vi "Save Recall Sweep List.vi"(8 "error in (no error)":errorcluster, 9 "File Name (\"\")":string, 10 "Sweep List Operation (0: Save)":u16(ring) items=["Save", "Recall"], 11 "VISA resource name":refnum<visa-resource-name>) -> (0 "error out":errorcluster, 3 "VISA resource name out":refnum<visa-resource-name>)   [LabVIEW 2009, in "Agilent PSG MXG Series.lvlib"]
doc: "Saves or recalls a sweep list to or from the file you specify."
uses:
  Agilent PSG MXG Series.lvlib
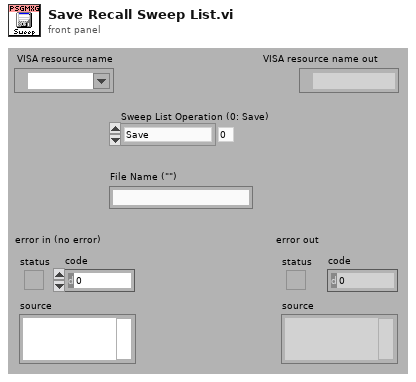
[diagram p1: front panel]
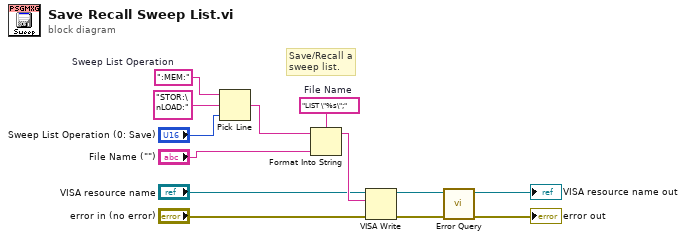
[diagram p0: block diagram]
diagram:
  w9 = "LIST \"%s\";"  # File Name
  w13 = ":MEM:"  # Sweep List Operation
  # "Save/Recall a\nsweep list."
  n1 = Pick Line(string ("")=w13, multi-line string="STOR:\nLOAD:", line index="Sweep List Operation (0: Save)") -> (output string=w10:string)
  n2 = Format Into String(format string=w9, initial string=w10, "File Name (\"\")") -> (resulting string=w7:string)  [unwired: 1 in, 1 out]
  n3 = VISA Write(VISA resource name="VISA resource name", write buffer=w7, error in (no error)="error in (no error)") -> (VISA resource name out=w6:refnum<visa-resource-name>, error out=w5:errorcluster)  [unwired: 1 out]
  n4 = call "Error Query.vi"("error in (no error)"=w5, "VISA resource name"=w6) -> ("error out"=→"error out":errorcluster, "VISA resource name out"=→"VISA resource name out":refnum<visa-resource-name>)  [unwired: 8 out]
